vi "Measure Voltage.vi"(8 "error in":errorcluster, 11 "BKPrecision in":refnum<class "9115AT.lvclass">) -> (0 "error out":errorcluster, 2 "Voltage":dbl, 3 "BKPrecision out":refnum<class "9115AT.lvclass">)   [LabVIEW 2018, in "9115AT.lvlib" / "9115AT.lvclass"]
uses:
  9115AT.lvclass
  builds/Power_Supply.lvlibp/Power Supply.lvclass
  <instrlib>/BK Precision 911X Series/BK Precision 911X Series.lvlib
  C:/Users/Ron.Dexter.LUMINARTECH/Desktop/builds/Power_Supply.lvlibp/Power Supply.lvclass
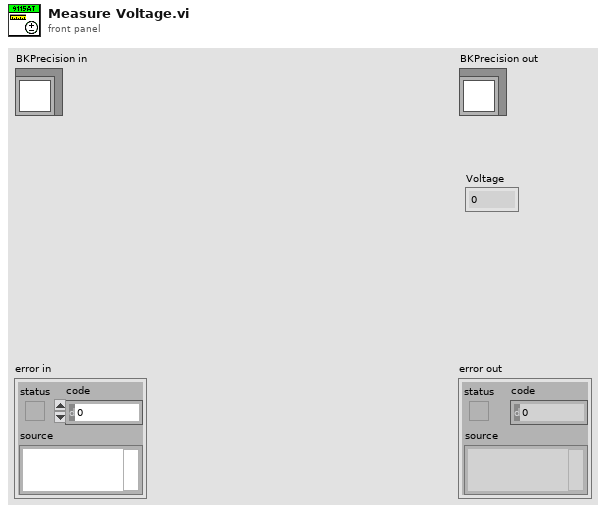
[diagram p1: front panel]
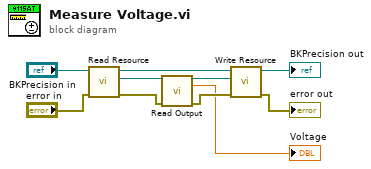
[diagram p0: block diagram]
diagram:
  n1 = call "Read Resource.vi"("error in"="error in", "Power Supply in"="BKPrecision in") -> ("error out"=w3:errorcluster, "Resource"=w5:refnum<visa-resource-name>, "Power Supply out"=w9:refnum<class "9115AT.lvclass">)  [unwired: 7 in]
  n2 = call <instrlib>:"Read Output.vi"("VISA resource name"=w5, "error in (no error)"=w3) -> ("VISA resource name out"=w4:refnum<visa-resource-name>, "Actual Voltage Level (V)"=→"Voltage":dbl, "error out"=w2:errorcluster)  [unwired: 8 in, 3 out]
  n3 = call "Write Resource.vi"("error in"=w2, "Resource"=w4, "Power Supply in"=w9) -> ("error out"=→"error out":errorcluster, "Power Supply out"=→"BKPrecision out":refnum<class "9115AT.lvclass">)  [unwired: 7 in]
